vi "DeleteSubscriber.vi"(8 "ErrorIn":errorcluster, 9 "TraceQueue":refnum<queue>, 11 "ITAFFilteredTrace in":refnum<class "ITAFFilteredTrace.lvclass">) -> (0 "ErrorOut":errorcluster, 3 "ITAFFilteredTrace out":refnum<class "ITAFFilteredTrace.lvclass">)   [LabVIEW 2021, in "ITAFFilteredTrace.lvclass"]
uses:
  ITAFFilteredTrace.lvclass
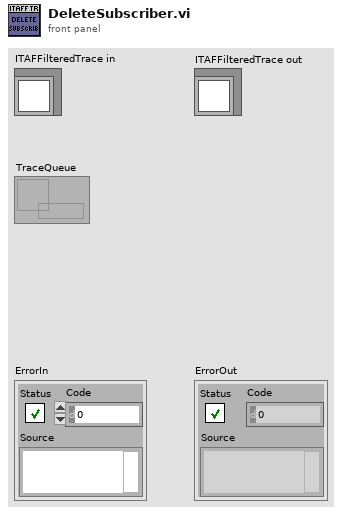
[diagram p1: front panel]
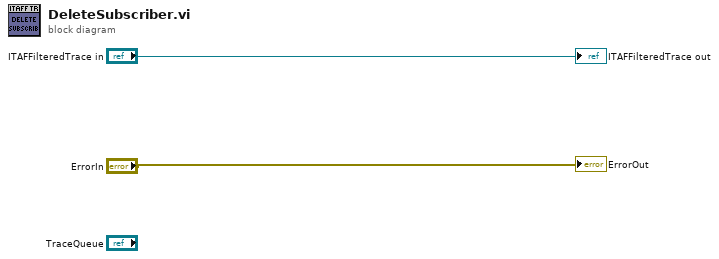
[diagram p0: block diagram]
diagram:
  "ErrorOut" <- "ErrorIn"
  "ITAFFilteredTrace out" <- "ITAFFilteredTrace in"
